vi "Working Thread.vi"(7 "EngineCSM":string, 10 "SocketName":string, 11 "Sequence":string) -> ()   [LabVIEW 2020, in "CSMScript-Engine(Lite).lvlib"]
uses:
  CSMScript-Engine(Lite).lvlib
  Typedef/Def-Thread Data.ctl
  Typedef/Def-StepComplete Event Data.ctl
  162d78b0-f25f-4e28-9f32-62a227129c30.vi
  3235fbb5-1003-4f8d-8a8e-733f49405df1.vi
  29c90474-5633-4ebd-9475-c7049fde7730.vi
  07558781-58e1-4dd2-b95a-dcbf6018b6a4.vi
  <userlib>/_NEVSTOP/Communicable State Machine(CSM)/AdvanceAPI/CSM - Set Module Attribute.vi
  <userlib>/_NEVSTOP/Communicable State Machine(CSM)/addons/API-String-Arugments-Support/_Support/Data To API String Arguments.vi
  <userlib>/_NEVSTOP/Communicable State Machine(CSM)/AdvanceAPI/CSM - Get Module Attribute.vi
  <userlib>/_NEVSTOP/Communicable State Machine(CSM)/Communicable State Machine.lvlib
  <userlib>/_NEVSTOP/Communicable State Machine(CSM)/_Shared/CSM Shared.lvlib
  <userlib>/_NEVSTOP/Communicable State Machine(CSM)/addons/API-String-Arugments-Support/API String Arguments Support.lvlib
panel:
  in  "Debug Stop":bool
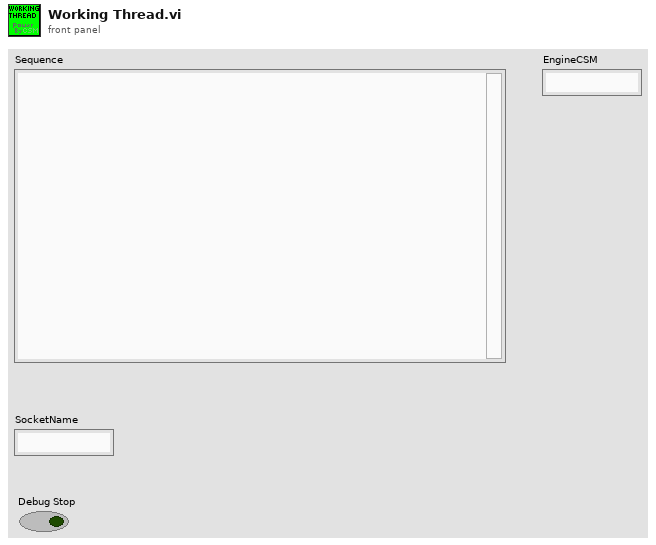
[diagram p1: front panel]
types:
  T1 = typedef "CSMScript-Engine(Lite).lvlib/Def-Thread Data.ctl" = cluster{"AUTO_ERROR_HANDLE":cluster{"ENABLE":bool, "ANCHOR":string}}
  T2 = typedef "CSMScript-Engine(Lite).lvlib/Def-StepComplete Event Data.ctl" = cluster{"index":i32, "Arguments":string, "error":errorcluster}
  T3 = cluster{"state":string, "args":string, "source/target":string}
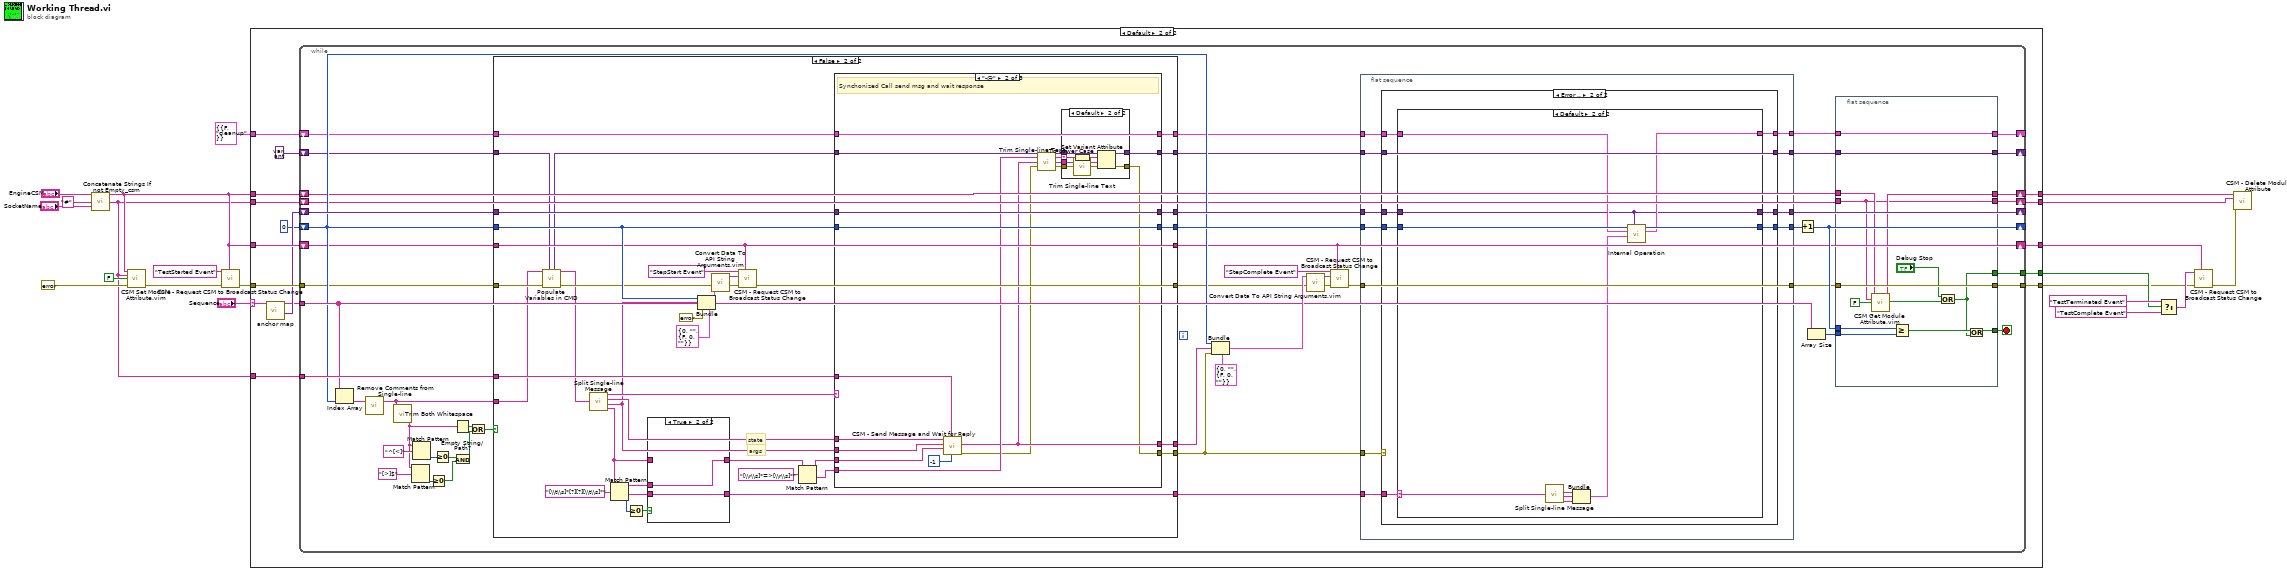
[diagram p0: block diagram]
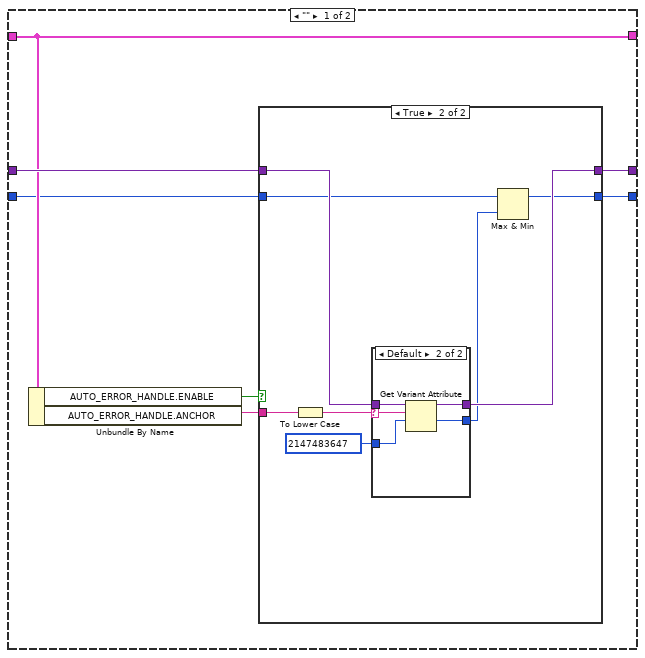
[diagram p4: hidden frame]
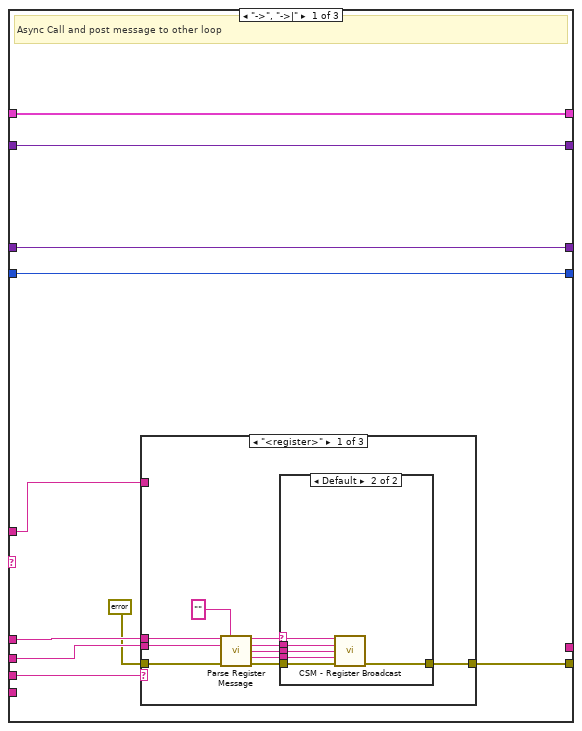
[diagram p9: hidden frame]
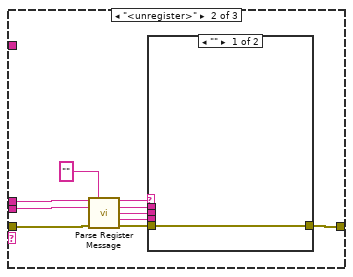
[diagram p11: hidden frame]
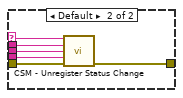
[diagram p12: hidden frame]
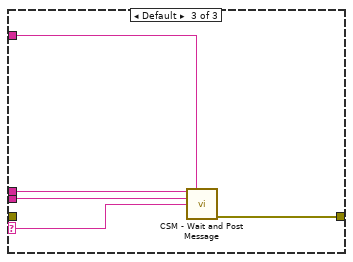
[diagram p13: hidden frame]
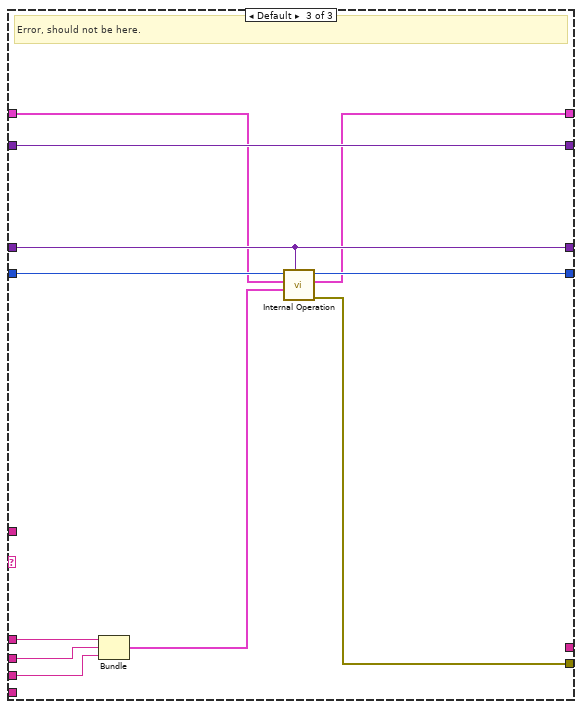
[diagram p15: hidden frame]
diagram:
  n1 = call <userlib>:"Concatenate Strings If not Empty_csm.vi"("String"="SocketName", "seperator(:)"="#", "prefix"="EngineCSM") -> ("result"=w2:string)  [unwired: 2 in]
  n2 = call "CSM Set Module Attribute.vim"("CSM Name"="EngineCSM", "Attribute"=w2, "Value"=FALSE, "Error In"=errorcluster {"status"=FALSE, "code"=0, "source"=""} ("error in (no error)")) -> ("error out"=w6:errorcluster)  [unwired: 8 in, 3 out]
  n3 = call <userlib>:"CSM - Request CSM to Broadcast Status Change.vi"("Module Name"="EngineCSM", "Error In (No Error)"=w6, "Status"="TestStarted Event") -> ("error out"=w19:errorcluster)  [unwired: 8 in]
  n4 = case shown="Default" "Sequence" {
    selector: "Sequence" -> [_ w34]
    tunnel: w19 -> [w23 w40]
    tunnel: "EngineCSM" -> [w24 w39]
    tunnel: [w24 w38] -> w18
    tunnel: [w23 w37] -> w10
    tunnel: w2 -> [_ w36]
    tunnel: "EngineCSM" -> [w22 w31]
    tunnel: [w22 w30] -> w13
    tunnel: [_ w29] -> w11
    tunnel: w2 -> [w21 w28]
    tunnel: [w21 w27] -> w7
    tunnel: T1 {"AUTO_ERROR_HANDLE"={"ENABLE"=FALSE, "ANCHOR"="cleanup"}} ("ThreadData") -> [_ w25]
    frame "False" {
    }
    frame Default {
      n5 = call "anchor map.vi"("string"=w34) -> ("Archt Map"=w35:variant, "Lines"=w33:string[])  [unwired: 9 in]
      n6 = while {
        tunnel: w40 -> [w54]
        tunnel: [w84] -> w37
        shift-right: [w51] -> w38
        shift-left: w39 -> [w52]
        tunnel: w36 -> [w91]
        tunnel: w33 -> [w81]
        shift-right: [w82] -> _
        shift-left: 0 -> [w58]
        shift-right: [w72] -> _
        shift-left: w35 -> [w79]
        shift-right: [w56] -> w30
        shift-left: w31 -> [w57]
        tunnel: [w55] -> w29
        shift-right: [w49] -> w27
        shift-left: w28 -> [w50]
        shift-right: [w48] -> _
        shift-left: variant -> [w45]
        shift-right: [w41] -> _
        shift-left: w25 -> [w44]
        stop <- w85 stop-if-true
        n7 = Index Array(array=w81, index=w58) -> (element=w83:string)
        n8 = call <userlib>:"Remove Comments from Single-line.vi"("single-line text"=w83) -> ("single-line text without comments"=w63:string)  [unwired: 2 in]
        n9 = call <userlib>:"Trim Both Whitespace.vi"("String"=w63) -> ("Trimmed String"=w62:string)  [unwired: 1 in]
        n10 = Match Pattern(string=w62, regular expression="[>]$") -> (offset past match=w68:i32)  [unwired: 1 in, 3 out]
        n11 = Match Pattern(string=w62, regular expression="^[<]") -> (offset past match=w69:i32)  [unwired: 1 in, 3 out]
        n12 = Greater Or Equal To 0?(x=w68) -> (x >= 0?=w67:bool)
        n13 = Greater Or Equal To 0?(x=w69) -> (x >= 0?=w66:bool)
        n14 = Empty String/Path?(string/path=w62) -> (empty?=w64:bool)
        n15 = And(x=w66, y=w67) -> (x .and. y?=w65:bool)
        n16 = Or(x=w64, y=w65) -> (x .or. y?=w61:bool)
        n17 = case shown="False" w61 {
          tunnel: w91 -> [_ w204]
          tunnel: [_ w203] -> w75
          tunnel: [_ w202] -> w87
          tunnel: [w168 w201] -> w59
          tunnel: w58 -> [w168 w184]
          tunnel: w79 -> [w167 w200]
          tunnel: [_ w193] -> w74
          tunnel: [w167 w192] -> w73
          tunnel: w63 -> [_ w174]
          tunnel: w54 -> [w166 w176]
          tunnel: [w166 w188] -> w53
          tunnel: w52 -> [w165 w182]
          tunnel: [w165 w182] -> w51
          tunnel: [w164 w181] -> w46
          tunnel: w45 -> [w164 w172]
          tunnel: w44 -> [w163 w170]
          tunnel: [w163 w169] -> w43
          frame True {
          }
          frame False {
            # "args"
            # "state"
            n18 = call "Populate Variables in CMD.vi"("Variant"=w172, "Error in"=w176, "String might with variables"=w174) -> ("Error out"=w175:errorcluster, "String out"=w173:string, "Variant Out"=w171:variant)  [unwired: 4 in]
            n19 = call <userlib>:"Split Single-line Message.vi"("single-line text"=w173) -> ("operator"=w206:string, "state"=w205:string, "args"=w183:string, "source/target"=w195:string)  [unwired: 6 in]
            n20 = Match Pattern(string=w195, regular expression="[\\t\\s]*[?][?][\\t\\s]*" ("string")) -> (before substring=w198:string, after substring=w194:string, offset past match=w197:i32)  [unwired: 1 in, 1 out]
            n21 = Greater Or Equal To 0?(x=w197) -> (x >= 0?=w196:bool)
            n22 = case shown="True" w196 {
              tunnel: w198 -> [_ w209]
              tunnel: w195 -> [w207 _]
              tunnel: [w207 w209] -> w179
              tunnel: w194 -> [_ w208]
              tunnel: [_ w208] -> w193
              frame False {
              }
              frame True {
              }
            }
            n23 = Bundle(cluster=T2 {"index"=0, "Arguments"="", "error"={"status"=FALSE, "code"=0, "source"=""}} ("output cluster"), "index"=w184, "Arguments"=w183, "error"=errorcluster {"status"=FALSE, "code"=0, "source"=""}) -> (w186:T2)
            n24 = call "Convert Data To API String Arguments.vim"("error in (no error)"=w175, "Data"=w186) -> ("error out"=w190:errorcluster, "API String"=w189:string)  [unwired: 6 in]
            n25 = call <userlib>:"CSM - Request CSM to Broadcast Status Change.vi"("Module Name"=w182, "Error In (No Error)"=w190, "Arguments (\"\")"=w189, "Status"="StepStart Event") -> ("error out"=w188:errorcluster)  [unwired: 7 in]
            n26 = Match Pattern(string=w179, regular expression="[\\r\\s]*=>[\\r\\s]*") -> (before substring=w178:string, after substring=w177:string)  [unwired: 1 in, 2 out]
            n27 = case shown="\"-@\"" w206 {
              tunnel: w205 -> [w215 w270 w287]
              tunnel: w183 -> [w214 w269 w286]
              tunnel: w204 -> [w216 w271 _]
              tunnel: w178 -> [w213 w268 w285]
              tunnel: [w217 w259 w290] -> w203
              tunnel: [_ w262 _] -> w202
              tunnel: [w219 w266 w292] -> w201
              tunnel: w184 -> [w219 w266 w291]
              tunnel: w200 -> [w218 w265 w289]
              tunnel: [w218 w265 w289] -> w192
              tunnel: [w211 w258 w288] -> w181
              tunnel: w171 -> [w211 w261 w288]
              tunnel: w177 -> [_ w263 _]
              tunnel: w170 -> [w210 w257 w283]
              tunnel: [w210 w257 w282] -> w169
              frame "->", "->|" {
                # "Async Call and post message to other loop"
                n28 = case shown="\"<register>\"" w213 {
                  selector: w213 -> [_ _ w256]
                  tunnel: w214 -> [w223 w239 w255]
                  tunnel: w215 -> [w224 w240 w254]
                  tunnel: errorcluster {"status"=FALSE, "code"=0, "source"=""} ("error IO") -> [w222 w238 _]
                  tunnel: [w221 w237 w252] -> w217
                  tunnel: w216 -> [_ _ w253]
                  frame "<register>" {
                    n29 = call <userlib>:"Parse Register Message.vi"("State"=w224, "Module Name"="", "Args"=w223) -> ("Target"=w228:string, "Source"=w227:string, "Status"=w226:string, "Api"=w225:string)  [unwired: 8 in, 1 out]
                    n30 = case shown="Default" w228 {
                      selector: w228 -> [_ w235]
                      tunnel: w227 -> [_ w234]
                      tunnel: w226 -> [_ w233]
                      tunnel: w225 -> [_ w232]
                      tunnel: w222 -> [w229 w231]
                      tunnel: [w229 w230] -> w221
                      frame "" {
                      }
                      frame Default {
                        n31 = call <userlib>:"CSM - Register Broadcast.vi"("CSM Name(Empty for Broadcast Event)"=w235, "Source CSM Name (* as Default)"=w234, "Trigger"=w233, "API (If \"\", Same as Trigger)"=w232, "Error In"=w231) -> ("error out"=w230:errorcluster)  [unwired: 9 in, 1 out]
                      }
                    }
                  }
                  frame "<unregister>" {
                    n32 = call <userlib>:"Parse Register Message.vi"("State"=w240, "Module Name"="", "Args"=w239) -> ("Target"=w244:string, "Source"=w243:string, "Status"=w242:string, "Api"=w241:string)  [unwired: 8 in, 1 out]
                    n33 = case shown="\"\"" w244 {
                      selector: w244 -> [_ w251]
                      tunnel: w243 -> [_ w250]
                      tunnel: w242 -> [_ w249]
                      tunnel: w241 -> [_ w248]
                      tunnel: w238 -> [w245 w247]
                      tunnel: [w245 w246] -> w237
                      frame "" {
                      }
                      frame Default {
                        n34 = call <userlib>:"CSM - Unregister Status Change.vi"("CSM Name"=w251, "Source CSM Name (* as Default)"=w250, "Status"=w249, "Response Message (\"*\" as Default)"=w248, "Error In"=w247) -> ("error out"=w246:errorcluster)  [unwired: 9 in, 1 out]
                      }
                    }
                  }
                  frame Default {
                    n35 = call <userlib>:"CSM - Wait and Post Message.vi"("State"=w254, "Current Module (\"\" to Generate an ID)"=w253, "Arguments (\"\")"=w255, "Target Module"=w256) -> ("error out"=w252:errorcluster)  [unwired: 10 in, 1 out]
                  }
                }
              }
              frame "-@" {
                # "Synchonized Call send msg and wait response"
                n36 = call <userlib>:"CSM - Send Message and Wait for Reply.vi"("Response Timeout (-2 Using Global Settings)"=-1 ("Response Timeout(5000ms)"), "Current Module (\"\" to Generate an ID)"=w271, "Target Module"=w268, "Arguments (\"\")"=w269, "State"=w270) -> ("error out"=w260:errorcluster, "Response"=w262:string)  [unwired: 4 in, 1 out]
                n37 = call <userlib>:"Trim Single-line Text.vi"("single-line text"=w263) -> ("trimed text"=w264:string)  [unwired: 2 in]
                n38 = case shown="Default" w264 {
                  selector: w264 -> [_ w279]
                  tunnel: w261 -> [w273 w281]
                  tunnel: [w273 w280] -> w258
                  tunnel: w262 -> [_ w278]
                  tunnel: [w272 w275] -> w259
                  tunnel: w260 -> [w272 w274]
                  frame "" {
                  }
                  frame Default {
                    n39 = To Lower Case(string=w279) -> (all lower case string=w276:string)
                    n40 = call <userlib>:"Trim Single-line Text.vi"("single-line text"=w278) -> ("trimed text"=w277:string)  [unwired: 2 in]
                    n41 = Set Variant Attribute(Variant=w281, name=w276, value=w277, error in=w274) -> (Variant out=w280:variant, error out=w275:errorcluster)  [unwired: 1 out]
                  }
                }
              }
              frame Default {
                # "Error, should not be here."
                n42 = Bundle("state"=w287, "args"=w286, "source/target"=w285) -> (w284:T3)  [unwired: 1 in]
                n43 = call "Internal Operation.vi"("Archt Map"=w289, "Message"=w284, "ThreadData"=w283, "Numeric in"=w291) -> ("error out"=w290:errorcluster, "ThreadData (dup)"=w282:T1, "Numeric out"=w292:i32)  [unwired: 5 in]
              }
            }
          }
        }
        n44 = Bundle(cluster=T2 {"index"=0, "Arguments"="", "error"={"status"=FALSE, "code"=0, "source"=""}} ("output cluster"), "index"=w58, "Arguments"=w87, "error"=w75) -> (w86:T2)
        n45 = call "Convert Data To API String Arguments.vim"("error in (no error)"=w53, "Data"=w86) -> ("error out"=w89:errorcluster, "API String"=w88:string)  [unwired: 6 in]
        n46 = call <userlib>:"CSM - Request CSM to Broadcast Status Change.vi"("Module Name"=w51, "Error In (No Error)"=w89, "Arguments (\"\")"=w88, "Status"="StepComplete Event") -> ("error out"=w77:errorcluster)  [unwired: 7 in]
        n47 = flat-sequence {
          tunnel: [w100] -> w78
          tunnel: w59 -> [w99]
          tunnel: w77 -> [w102]
          tunnel: [w102] -> w76
          tunnel: w75 -> [w101]
          tunnel: w74 -> [w98]
          tunnel: w73 -> [w97]
          tunnel: [w96] -> w72
          tunnel: [w95] -> w47
          tunnel: w46 -> [w94]
          tunnel: w43 -> [w93]
          tunnel: [w92] -> w42
          frame #0 {
            n48 = case shown="Error .." w101 {
              tunnel: [w106 w113] -> w100
              tunnel: w99 -> [w106 w114]
              tunnel: w98 -> [_ w112]
              tunnel: w97 -> [w105 w111]
              tunnel: [w105 w107] -> w96
              tunnel: [w104 w110] -> w95
              tunnel: w94 -> [w104 w110]
              tunnel: w93 -> [w103 w109]
              tunnel: [w103 w108] -> w92
              frame No Error {
              }
              frame Error {
                n49 = case shown="Default" w112 {
                  selector: w112 -> [_ w146]
                  tunnel: w114 -> [w116 w148]
                  tunnel: [w115 w147] -> w113
                  tunnel: w111 -> [w121 w139]
                  tunnel: w109 -> [w119 w141]
                  tunnel: [w119 w140] -> w108
                  tunnel: [w120 w139] -> w107
                  frame "" {
                    n50 = Unbundle By Name(w119) -> ("AUTO_ERROR_HANDLE.ENABLE"=w117:bool, "AUTO_ERROR_HANDLE.ANCHOR"=w118:string)
                    n51 = case shown="True" w117 {
                      tunnel: w121 -> [w123 w130]
                      tunnel: [w123 w129] -> w120
                      tunnel: w118 -> [_ w128]
                      tunnel: w116 -> [w122 w125]
                      tunnel: [w122 w124] -> w115
                      frame False {
                      }
                      frame True {
                        n52 = To Lower Case(string=w128) -> (all lower case string=w131:string)
                        n53 = case shown="Default" w131 {
                          selector: w131 -> [_ w138]
                          tunnel: w130 -> [w133 w137]
                          tunnel: [w133 w136] -> w129
                          tunnel: [w132 w135] -> w126
                          tunnel: 2147483647 -> [w132 w134]
                          frame "" {
                          }
                          frame Default {
                            n54 = Get Variant Attribute(Variant=w137, name=w138, default value (empty Variant)=w134) -> (duplicate Variant=w136:variant, value=w135:i32)  [unwired: 1 in, 2 out]
                          }
                        }
                        n55 = Max & Min(x=w125, y=w126) -> (max(x,y)=w124:i32)  [unwired: 1 out]
                      }
                    }
                  }
                  frame Default {
                    n56 = call <userlib>:"Split Single-line Message.vi"("single-line text"=w146) -> ("state"=w145:string, "args"=w144:string, "source/target"=w143:string)  [unwired: 6 in, 1 out]
                    n57 = Bundle("state"=w145, "args"=w144, "source/target"=w143) -> (w142:T3)  [unwired: 1 in]
                    n58 = call "Internal Operation.vi"("Archt Map"=w139, "Message"=w142, "ThreadData"=w141, "Numeric in"=w148) -> ("ThreadData (dup)"=w140:T1, "Numeric out"=w147:i32)  [unwired: 5 in, 1 out]
                  }
                }
              }
            }
          }
        }
        n59 = Increment(x=w78) -> (x+1=w82:i32)
        n60 = Array Size(array=w81) -> (size(s)=w80:i32)
        n61 = flat-sequence {
          tunnel: [w162] -> w85
          tunnel: [w161] -> w84
          tunnel: w76 -> [w161]
          tunnel: w82 -> [w159]
          tunnel: w80 -> [w158]
          tunnel: w57 -> [w157]
          tunnel: [w156] -> w56
          tunnel: [w154] -> w55
          tunnel: w50 -> [w151]
          tunnel: [w151] -> w49
          tunnel: [w150] -> w48
          tunnel: w47 -> [w150]
          tunnel: w42 -> [w149]
          tunnel: [w149] -> w41
          frame #0 {
            n62 = call "CSM Get Module Attribute.vim"("CSM Name"=w157, "Attribute"=w151, "Default Value (Empty Variant)"=FALSE) -> ("CSM Name (Dup)"=w156:string, "Value"=w153:bool)  [unwired: 8 in, 3 out]
            n63 = Greater Or Equal?(x=w159, y=w158) -> (x >= y?=w160:bool)
            n64 = Or(x="Debug Stop", y=w153) -> (x .or. y?=w154:bool)
            n65 = Or(x=w160, y=w154) -> (x .or. y?=w162:bool)
          }
        }
      }
    }
  }
  n66 = Select(t="TestTerminated Event" ("Status"), s=w11, f="TestComplete Event" ("Status")) -> (s? t:f=w17:string)
  n67 = call <userlib>:"CSM - Request CSM to Broadcast Status Change.vi"("Module Name"=w18, "Error In (No Error)"=w10, "Status"=w17) -> ("error out"=w12:errorcluster)  [unwired: 8 in]
  n68 = call <userlib>:"CSM - Delete Module Attribute.vi"("CSM Name"=w13, "Attribute"=w7, "Error In"=w12) -> ()  [unwired: 9 in, 4 out]
